vi "Auton go linear distance.vi"(0 "Average gains":T1, 1 "PID setpoint":dbl, 2 "Goal":dbl, 4 "output range":cluster{"output high":dbl, "output low":dbl}) -> (5 "Done?":bool)   [LabVIEW 2014]
uses:
  DriveGlobal.vi
  <vilib>/addons/control/pid/pid.llb/PID (DBL).vi
  Robot Values.vi
  <vilib>/addons/control/pid/NI_PID_pid.lvlib
panel:
  in  "Diffrence gains":T1={"proportional gain (Kc)"=0.01, "integral time (Ti, min)"=0.0, "derivative time (Td, min)"=0.0} {"derivative time (Td, min)" format="%.3f"; "integral time (Ti, min)" format="%.3f"; "proportional gain (Kc)" format="%.3f"}
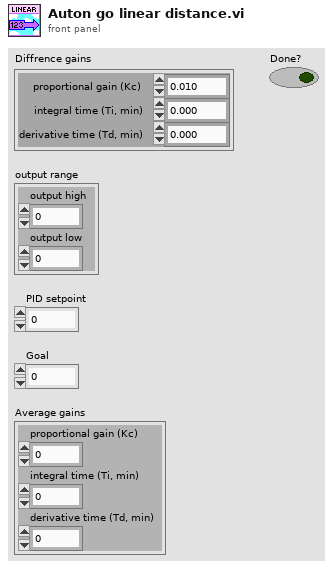
[diagram p1: front panel]
types:
  T1 = cluster{"proportional gain (Kc)":dbl, "integral time (Ti, min)":dbl, "derivative time (Td, min)":dbl}
  T2 = cluster{"Tracking Tote?":bool, "ToteRightSpeed":dbl, "ToteLeftSpeed":dbl, "Drive Encoder reset":bool, "Right Wheel \n(Cm)":dbl, "Left Wheel \n(Cm)":dbl}
  T3 = cluster{"RightMotorSpeed":dbl, "LeftMotorSpeed":dbl}
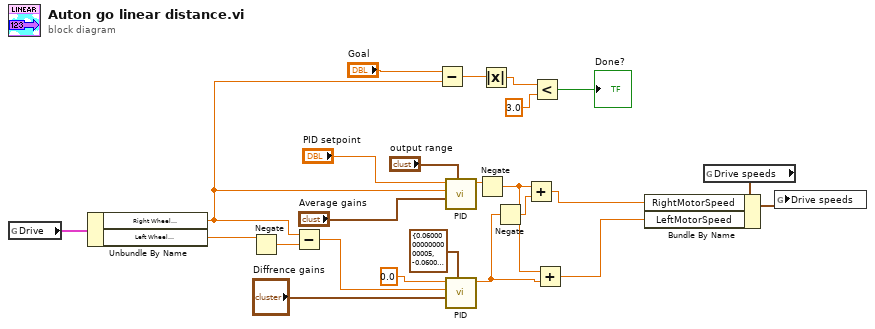
[diagram p0: block diagram]
diagram:
  n1 = global read "Robot Values.vi" "Drive"() -> (w20:T2)
  n2 = Unbundle By Name(w20) -> ("Right Wheel \n(Cm)"=w6:dbl, "Left Wheel \n(Cm)"=w23:dbl)
  n3 = Negate(x=w23) -> (-x=w10:dbl)
  n4 = Subtract(x=w6, y=w10) -> (x-y=w11:dbl)
  n5 = Subtract(x="Goal", y=w6) -> (x-y=w5:dbl)
  n6 = call-poly <vilib>:"PID.vi"("output range"="output range", "PID gains"="Average gains", "process variable"=w6, "setpoint"="PID setpoint") -> ("output"=w15:dbl)  [unwired: 6 in, 1 out]
  n7 = call-poly <vilib>:"PID.vi"("output range"=cluster{"output high":dbl, "output low":dbl} {"output high"=0.060000000000000005, "output low"=-0.060000000000000005}, "PID gains"="Diffrence gains", "process variable"=w11, "setpoint"=0.0) -> ("output"=w16:dbl)  [unwired: 6 in, 1 out]
  n8 = Negate(x=w15) -> (-x=w18:dbl)
  n9 = Absolute Value(x=w5) -> (abs(x)=w4:dbl)
  n10 = Negate(x=w16) -> (-x=w17:dbl)
  n11 = Add(x=w18, y=w17) -> (x+y=w21:dbl)
  n12 = Less?(x=w4, y=3.0) -> (x < y?=→"Done?":bool)
  n13 = Add(x=w18, y=w16) -> (x+y=w22:dbl)
  n14 = global read "DriveGlobal.vi" "Drive speeds"() -> (w7:T3)
  n15 = Bundle By Name(cluster=w7, "RightMotorSpeed"=w21, "LeftMotorSpeed"=w22) -> (w8:T3)
  n16 = global write "DriveGlobal.vi" "Drive speeds"(w8) -> ()
